vi "Get Transceiver Threads.vi"(11 "Plugin in":refnum<class "Plugin.lvclass">) -> (2 "Transceiver Threads":refnum<class "Transceiver Interface.lvclass">[](array[class]), 3 "Plugin out":refnum<class "Plugin.lvclass">)   [LabVIEW 2017, in "Data Sharing Framework Core.lvlib" / "Data Sharing Framework Engine.lvlib" / "Plugin.lvclass"]
uses:
  Plugin.lvclass
  Internal/Interfaces/Transceiver Interface/Transceiver Interface.lvclass
  Plugin.lvclass/Plugin.ctl
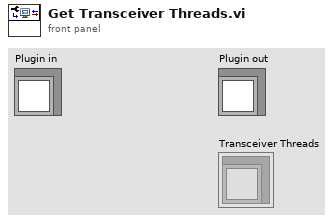
[diagram p1: front panel]
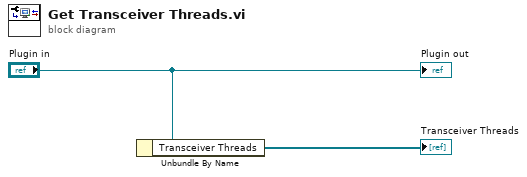
[diagram p0: block diagram]
diagram:
  n1 = Unbundle By Name("Plugin in") -> ("Transceiver Threads"=→"Transceiver Threads":refnum<class "Transceiver Interface.lvclass">[])
  "Plugin out" <- "Plugin in"
